vi "SelectOperation-TernaryOps.vi"() -> ()   [LabVIEW 2019]
panel:
  out "var":string
  in  "a":dbl
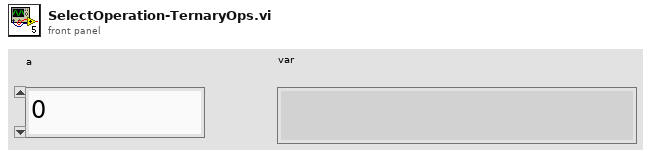
[diagram p1: front panel]
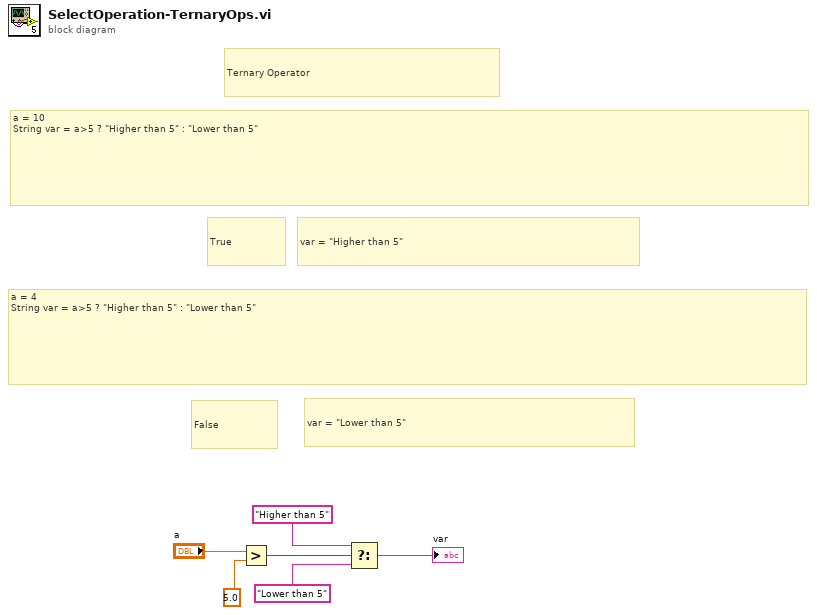
[diagram p0: block diagram]
diagram:
  # "var = \"Lower than 5\""
  # "False"
  # "a = 4\nString var = a>5 ? \"Higher than 5\" : \"Lower than 5\""
  # "var = \"Higher than 5\""
  # "True"
  # "a = 10\nString var = a>5 ? \"Higher than 5\" : \"Lower than 5\""
  # "Ternary Operator"
  n1 = Greater?(x="a", y=5.0) -> (0:w4:bool)
  n2 = Select(t="Higher than 5", s=w4, f="Lower than 5") -> (s? t:f=→"var":string)
